vi "State Space Modeling.vi"() -> ()   [LabVIEW 2019]
uses:
  <vilib>/Simulation/Scripting/Companion Diagram/SimConfigNode/SimParams.ctl
  <vilib>/Simulation/Scripting/Companion Diagram/SimConfigNode/_simSolvers.ctl
  <vilib>/Simulation/Implementation/Shared/SIMSCR Execution Mode.ctl
  <vilib>/Platform/TimedLoop/XDataNode/timing_clust.ctl
  <vilib>/Platform/TimedLoop/XDataNode/nitl_modes.ctl
  <vilib>/Platform/TimedLoop/XDataNode/wakeup.ctl
  <vilib>/Simulation/Param Hierarchy/Typedefs/SIMPH Param Control Actions.ctl
  <vilib>/Simulation/Implementation/Shared/NILVSim_ParamChanged.vi
  <vilib>/Simulation/Implementation/Shared/NILVSim_FinishedLate.vi
  <vilib>/Simulation/Implementation/Shared/NILVSIM_BeginStep.vi
  <vilib>/Simulation/Utility/Implementation/SIM Halt.vi
  <vilib>/Simulation/DataSources/Implementation/NILVSim Signal Generator.llb/SIM Signal Generator (scalar).vi
  <vilib>/Simulation/SignalArithmetic/Implementation/NILVSim Gain.llb/SIM Gain (scalar).vi
  <vilib>/Simulation/Nonlinear/Implementation/NILVSim Saturation.llb/SIM Saturation (scalar).vi
  <vilib>/Simulation/ContinuousLinear/Implementation/NILVSim State Space.llb/SIM State Space Distributor (CD).vi
  <vilib>/Simulation/ContinuousLinear/Implementation/NILVSim State Space.llb/SIM State Space Collector (CD).vi
  <vilib>/Simulation/Implementation/Shared/NILVSim_Manager.vi
  <vilib>/Utility/error.llb/Clear Errors.vi
  <vilib>/Simulation/Implementation/Shared/NILVSim_FinalizeModel.vi
  <vilib>/imath/engines/lvmath2/RunTimeEngine/IndexRead/NIMS M(S,S).vi
  <instcachedir>/0/NIMS M(S,S)_AC51E74150A542F7991B9634C66F3096.lvgen/NIMS M(S,S)_AC51E74150A542F7991B9634C66F3096_002.vi
  <vilib>/imath/engines/lvmath2/RunTimeEngine/IndexRead/NIMS V(S).vi
  <instcachedir>/0/NIMS V(S)_0488751826AF41519A22953C041130DC.lvgen/NIMS V(S)_0488751826AF41519A22953C041130DC_000.vi
  <vilib>/imath/engines/lvmath2/RunTimeEngine/IndexReplace/NIMS M(S,S)=S.vi
  <instcachedir>/0/NIMS M(S,S)=S_F60428D0350A4667AE68E0C0372F4DD1.lvgen/NIMS M(S,S)=S_F60428D0350A4667AE68E0C0372F4DD1_000.vi
  <vilib>/imath/engines/lvmath2/RunTimeEngine/ErrorHandling/NIMS_Create Error From Enums.vi
  <instcachedir>/0/NIMS M(S,S)_AC51E74150A542F7991B9634C66F3096.lvgen/NIMS M(S,S)_AC51E74150A542F7991B9634C66F3096_000.vi
  <vilib>/imath/engines/lvmath/Plug In/Control Design/BuiltInFunctions/ss/NIMS_CD_ss(A,B,C,D).vi
  <vilib>/imath/engines/lvmath2/RunTimeEngine/NodeEndStatement/NIMS_NodeEndStatement_Output.vi
  <instcachedir>/0/NIMS_NodeEndStatement_Output_53EC0D466D134D7ABD903AC30B43404B.lvgen/NIMS_NodeEndStatement_Output_53EC0D466D134D7ABD903AC30B43404B_010.vi
  <vilib>/imath/engines/lvmath2/RunTimeEngine/ErrorHandling/NIMS_Finalize Error.vi
  <vilib>/Simulation/Implementation/Shared/SIM Unbundle Sim Info.vi
  <vilib>/Simulation/Implementation/Shared/SIMSH Read Queue.vi
  <vilib>/Simulation/Implementation/Shared/NILVSim_Initialize.vi
  <vilib>/Simulation/Utility/Implementation/NILVSim Get Time and IsAcceptedStep.vi
  SubVIs/Motor.vi
  SubVIs/Encoders.vi
  <vilib>/Simulation/Implementation/Shared/NILVSim_GetModelError.vi
  <vilib>/Simulation/Implementation/Shared/SIM Bundle Sim Info.vi
  <vilib>/addons/Control Design/_Utility/Model Viewer.llb/Model Viewer SubVI/cd_Draw State-Space Equation (SS).vi
  <vilib>/Simulation/Scripting/Companion Diagram/SimConfigNode/SimDog.xnode
  <vilib>/addons/Control Design/_Model Construction/Model Typedefs.llb/CD State Space Model (MIMO).ctl
  <vilib>/addons/Control Design/_Model Construction/Model Typedefs.llb/CD General Elements.ctl
  <vilib>/Platform/TimedLoop/XDataNode/XDataNode.xnode
  <vilib>/Simulation/Implementation/XNodeFramework/SimXNode/SimX.xnode
  <vilib>/addons/Control Design/_Model Construction/NI_LinSys_Model Typedefs.lvlib
  <vilib>/addons/Control Design/_Utility/NI_CD_Model Viewer.lvlib
  <vilib>/Simulation/ContinuousLinear/Implementation/NILVSim State Space.llb/SIM State Space (CD).vi
  <vilib>/Platform/TimedLoop/XDataNode/XDNodeRunTimeDep.lvlib
  <vilib>/Simulation/Implementation/Shared/NI_SIM_Implementation.lvlib
panel:
  out "Open Loop State-Space Model":picture
  in  "Stop Button":bool
  in  "Motor Parameters":T1={"Rm (ohm)"=8.4, "km (V-s/rad)"=0.042, "kt (N-m/A)"=0.042} {"kt (N-m/A)" min=0.0 format="%_3g"; "km (V-s/rad)" min=0.0 format="%_3g"; "Rm (ohm)" min=0.0 format="%_3f"}
  in  "Pendulum Parameters":T2={"mp (kg)"=0.024, "Lr (m)"=0.085, "Lp (m)"=0.129, "Jr (kg.m^2)"=5.72e-05, "Dr (N.m.s/rad)"=0.0015, "Jp (kg.m^2)"=3.33e-05, "Dp (N.m.s/rad)"=0.0005, "g (m/s^2)"=9.81} {"g (m/s^2)" min=0.0 format="%_3g"; "Lr (m)" min=0.0 format="%_3g"; "Dr (N.m.s/rad)" min=0.0 format="%_3g"; "Jr (kg.m^2)" min=0.0 format="%_3g"; "Dp (N.m.s/rad)" min=0.0 format="%_3g"; "Jp (kg.m^2)" min=0.0 format="%_3g"; "Lp (m)" min=0.0 format="%_3g"; "mp (kg)" min=0.0 format="%_3f"}
  out "Pendulum Angle (rad)":cluster{"output":dbl, dbl}(graph)
  out "Rotary Arm Angle (rad)":cluster{"output":dbl, dbl}(graph)
  # "Controls Board"
  # "State-Space Modeling"
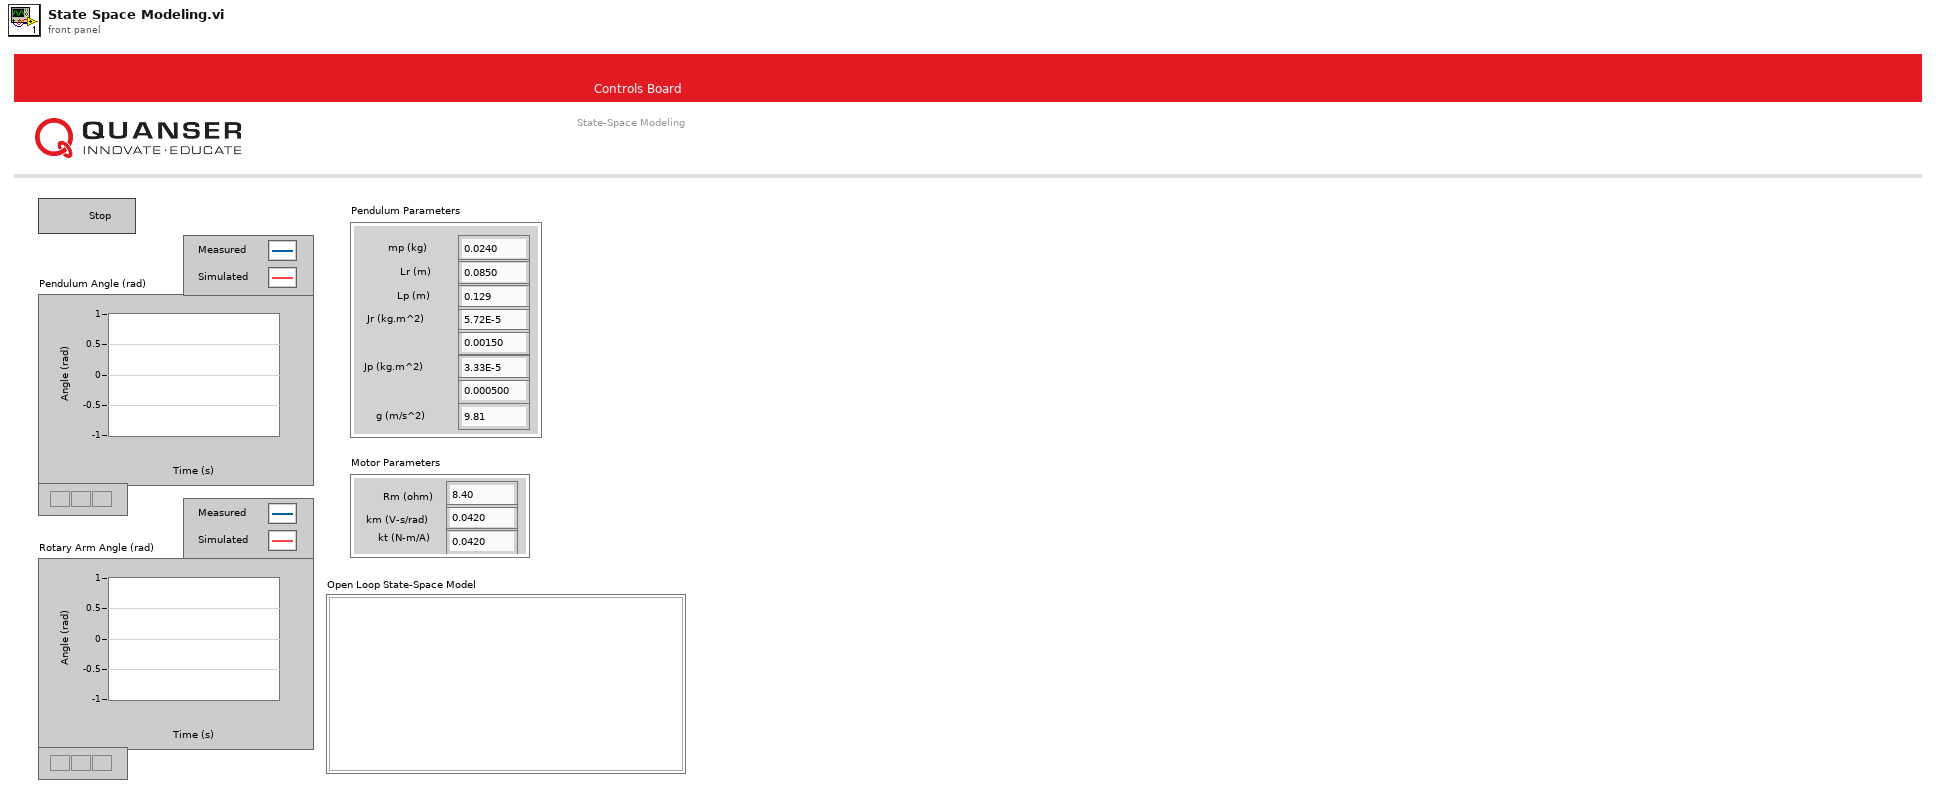
[diagram p1: front panel]
types:
  T1 = cluster{"Rm (ohm)":dbl, "km (V-s/rad)":dbl, "kt (N-m/A)":dbl}
  T2 = cluster{"mp (kg)":dbl, "Lr (m)":dbl, "Lp (m)":dbl, "Jr (kg.m^2)":dbl, "Dr (N.m.s/rad)":dbl, "Jp (kg.m^2)":dbl, "Dp (N.m.s/rad)":dbl, "g (m/s^2)":dbl}
  T3 = typedef "NI_LinSys_Model Typedefs.lvlib/CD State Space Model (MIMO).ctl" = cluster{"properties":T4, "A":dbl[][], "B":dbl[][], "C":dbl[][], "D":dbl[][], "StateNames":string[], "Transport Delay":dbl[][]}
  T4 = typedef "NI_LinSys_Model Typedefs.lvlib/CD General Elements.ctl" = cluster{"Model name":string, "Input names":string[], "Output names":string[], "Input Delays":dbl[], "Output Delays":dbl[], "Sampling Time":dbl, "Notes":string}
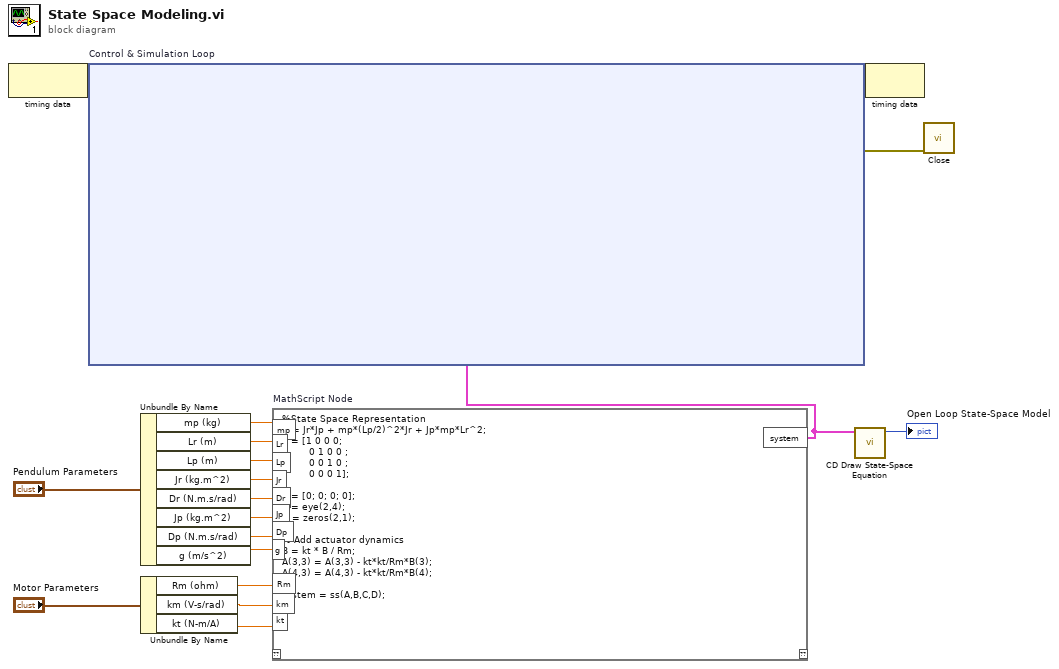
[diagram p0: block diagram]
diagram:
  n1 = node-c288() -> (w18:variant)  [unwired: 1 in]
  n2 = Unbundle By Name("Pendulum Parameters") -> ("mp (kg)"=w16:dbl, "Lr (m)"=w15:dbl, "Lp (m)"=w14:dbl, "Jr (kg.m^2)"=w13:dbl, "Dr (N.m.s/rad)"=w12:dbl, "Jp (kg.m^2)"=w11:dbl, "Dp (N.m.s/rad)"=w10:dbl, "g (m/s^2)"=w9:dbl)
  n3 = Unbundle By Name ("Unbundle By Name 2")("Motor Parameters") -> ("Rm (ohm)"=w8:dbl, "km (V-s/rad)"=w7:dbl, "kt (N-m/A)"=w6:dbl)
  n4 = mathscript code="%State Space Representation\nJt = Jr*Jp + mp*(Lp/2)^2*Jr + Jp*mp*Lr^2;\nA = [1 0 0 0;\n         0 1 0 0 ;\n         0 0 1 0 ;\n         0 0 0 1];\n\nB = [0; 0; 0; 0];\nC = eye(2,4);\nD = zeros(2,1);\n\n% Add actuator dynamics\nB = kt * B / Rm;\nA(3,3) = A(3,3) - kt*kt/Rm*B(3);\nA(4,3) = A(4,3) - kt*kt/Rm*B(4);\n\nsystem = ss(A,B,C,D);"("mp"=w16, "Lr"=w15, "Lp"=w14, "Jr"=w13, "Dr"=w12, "Jp"=w11, "Dp"=w10, "g"=w9, "kt"=w6, "km"=w7, "Rm"=w8) -> ("system"=w3:T3)  [unwired: 1 in, 1 out]
  n5 = node-c254 "Control & Simulation Loop"(w18, w3) -> (w17:variant, w1:errorcluster)
  n6 = call-poly <vilib>:"CD Draw State-Space Equation.vi"("State-Space Model"=w3) -> ("Equation"=→"Open Loop State-Space Model":picture)  [unwired: 8 in, 2 out]
  n7 = node-c288(w17) -> ()  [unwired: 1 out]
  n8 = call "Close.vi"("error in"=w1) -> ()  [unwired: 10 in, 1 out]
